vi "logToFile.vi"() -> ()   [LabVIEW 2017]
uses:
  <vilib>/Utility/file.llb/Write Delimited Spreadsheet (DBL).vi
panel:
  out "Elapsed time <s>":dbl format="%#_13g"
  in  "PWM Command":dbl min=0.0 max=255.0 step=1.0
  out "Voltage Chart":waveform(dbl)(graph)
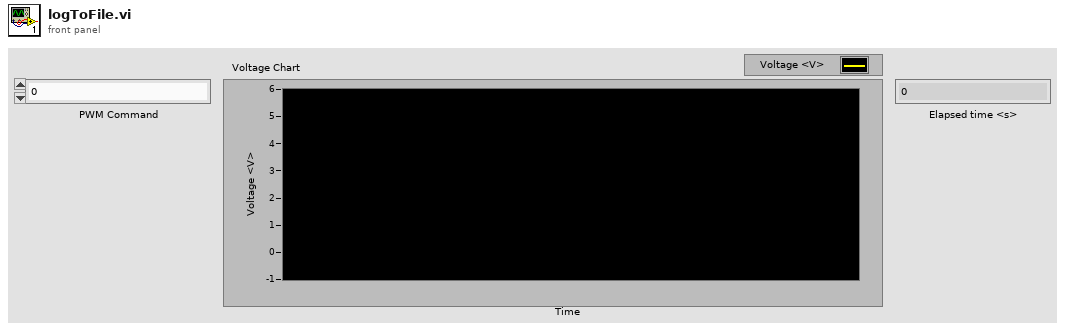
[diagram p1: front panel]
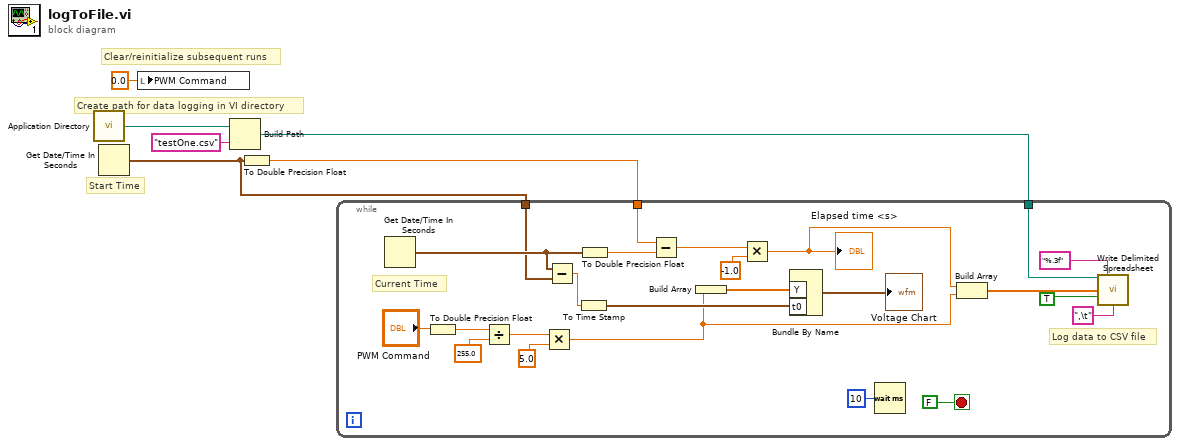
[diagram p0: block diagram]
diagram:
  # "Create path for data logging in VI directory"
  # "Clear/reinitialize subsequent runs"
  # "Start Time"
  n1 = call <vilib>:"Application Directory.vi"() -> ("Application Directory"=w1:path)
  n2 = Get Date/Time In Seconds() -> (seconds since 1Jan1904=w4:timestamp)
  n3 = local write "PWM Command"(0.0 ("PWM Command")) -> ()
  n4 = Build Path(base path=w1, name or relative path="testOne.csv") -> (appended path=w2:path)
  n5 = To Double Precision Float(number=w4) -> (double precision float=w5:dbl)
  n6 = while {
    tunnel: w5 -> [w24]
    tunnel: w4 -> [w16]
    tunnel: w2 -> [w7]
    stop <- FALSE stop-if-true
    # "Log data to CSV file"
    # "Current Time"
    n7 = Get Date/Time In Seconds() -> (seconds since 1Jan1904=w17:timestamp)
    n8 = To Double Precision Float(number="PWM Command") -> (double precision float=w25:dbl)
    n9 = Divide(x=w25, y=255.0) -> (x/y=w28:dbl)
    n10 = Multiply(x=w28, y=5.0) -> (x*y=w11:dbl)
    n11 = Subtract(x=w17, y=w16) -> (x-y=w15:dbl)
    n12 = To Time Stamp(1:w15) -> (0:w14:timestamp)
    n13 = To Double Precision Float(number=w17) -> (double precision float=w20:dbl)
    n14 = Subtract(x=w24, y=w20) -> (x-y=w23:dbl)
    n15 = Build Array(w11) -> (w19:dbl[])
    n16 = Multiply(x=w23, y=-1.0) -> (x*y=w12:dbl)
    "Elapsed time <s>" <- w12
    n17 = Bundle By Name("Y"=w19, "t0"=w14) -> (→"Voltage Chart":waveform(dbl))  [unwired: 1 in]
    n18 = Wait (ms)(milliseconds to wait=u32 10) -> ()  [unwired: 1 out]
    n19 = Build Array(w12, w11) -> (w10:dbl[])
    n20 = call-poly <vilib>:"Write Delimited Spreadsheet.vi"("file path (dialog if empty)"=w7, "format (%.3f)"="%.3f", "1D data"=w10, "append to file? (new file:F)"=TRUE, "delimiter (\\t)"=",\t" ("delimiter (\\t)")) -> ()  [unwired: 9 in, 2 out]
  }
